vi "SRX_Read Quad Sensor Data.vi"(8 "Error":errorcluster, 11 "PhoenixMotorControlDevRef":T2) -> (0 "Error Out":errorcluster, 3 "Quad Sensor Data Out":T1)   [LabVIEW 2017]
uses:
  <vilib>/Rock Robotics/WPI/MotorControl/WPI_MotorControlDeviceRef.ctl
  <vilib>/Rock Robotics/WPI/MotorControl/WPI_MotorControlType.ctl
  <vilib>/Rock Robotics/SystemInterfaces/DIO/FPGA_DIOPWMChannel.ctl
  <vilib>/Rock Robotics/WPI/PWM/WPI_PWMDeadband.ctl
  <vilib>/Rock Robotics/SystemInterfaces/DIO/FPGA_DIOChannel.ctl
  TypeDefs SRX/Cluster_SRX_Sensor Quad Data.ctl
  System Drivers/Phoenix-LabVIEW/Motor Controller/Get/CTRE_Phoenix_MotorController_GetQuadPinData.vi
  System Drivers/Phoenix-LabVIEW/Motor Controller/Get/CTRE_Phoenix_MotorController_GetQuadratureData.vi
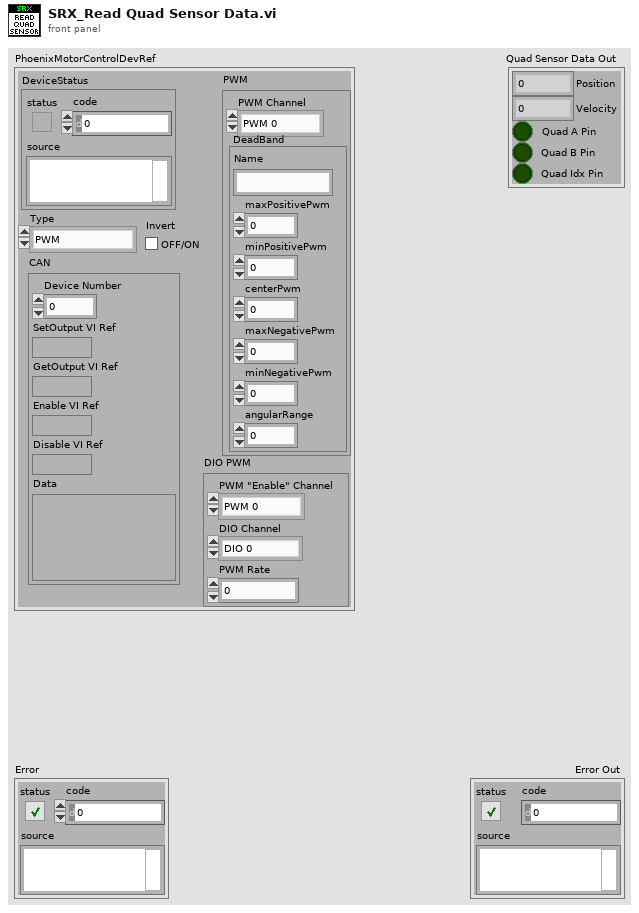
[diagram p1: front panel]
types:
  T1 = typedef "Cluster_SRX_Sensor Quad Data.ctl" = cluster{"Position":i32, "Velocity":i32, "Quad A Pin":bool, "Quad B Pin":bool, "Quad Idx Pin":bool}
  T2 = typedef "WPI_MotorControlDeviceRef.ctl" = cluster{"DeviceStatus":errorcluster, "Type":T3, "PWM":cluster{"PWM Channel":T4, "DeadBand":T5}, "CAN":cluster{"Device Number":u8, "SetOutput VI Ref":variant, "GetOutput VI Ref":variant, "Enable VI Ref":variant, "Disable VI Ref":variant, "Data":variant}, "Invert":bool, "DIO PWM":cluster{"PWM \"Enable\" Channel":T4, "DIOChannel":T6, "PWM Rate":dbl}}
  T3 = typedef "WPI_MotorControlType.ctl" = enum16{"PWM", "CAN", "DIO PWM"}
  T4 = typedef "FPGA_DIOPWMChannel.ctl" = enum8{"PWM 0", "PWM 1", "PWM 2", "PWM 3", "PWM 4", "PWM 5", "PWM 6", "PWM 7", "PWM 8", "PWM 9", "PWM MXP 0", "PWM MXP 1", "PWM MXP 2", "PWM MXP 3", "PWM MXP 4", "PWM MXP 5", "PWM MXP 6", "PWM MXP 7", "PWM MXP 8", "PWM MXP 9", "Invalid"}
  T5 = typedef "WPI_PWMDeadband.ctl" = cluster{"Name":string, "maxPositivePwm":i32, "minPositivePwm":i32, "centerPwm":i32, "maxNegativePwm":i32, "minNegativePwm":i32, "angularRange":u16}
  T6 = typedef "FPGA_DIOChannel.ctl" = enum8{"DIO 0", "DIO 1", "DIO 2", "DIO 3", "DIO 4", "DIO 5", "DIO 6", "DIO 7", "DIO 8", "DIO 9", "DIO MXP 0", "DIO MXP 1", "DIO MXP 2", "DIO MXP 3", "DIO MXP 4", "DIO MXP 5", "DIO MXP 6", "DIO MXP 7", "DIO MXP 8", "DIO MXP 9", "DIO MXP 10", "DIO MXP 11", "DIO MXP 12", "DIO MXP 13", "DIO MXP 14", "DIO MXP 15", "SPI Port CS1", "SPI Port CS2", "SPI Port CS3", "SPI Port MISO", "SPI Port MOSI", "Invalid"}
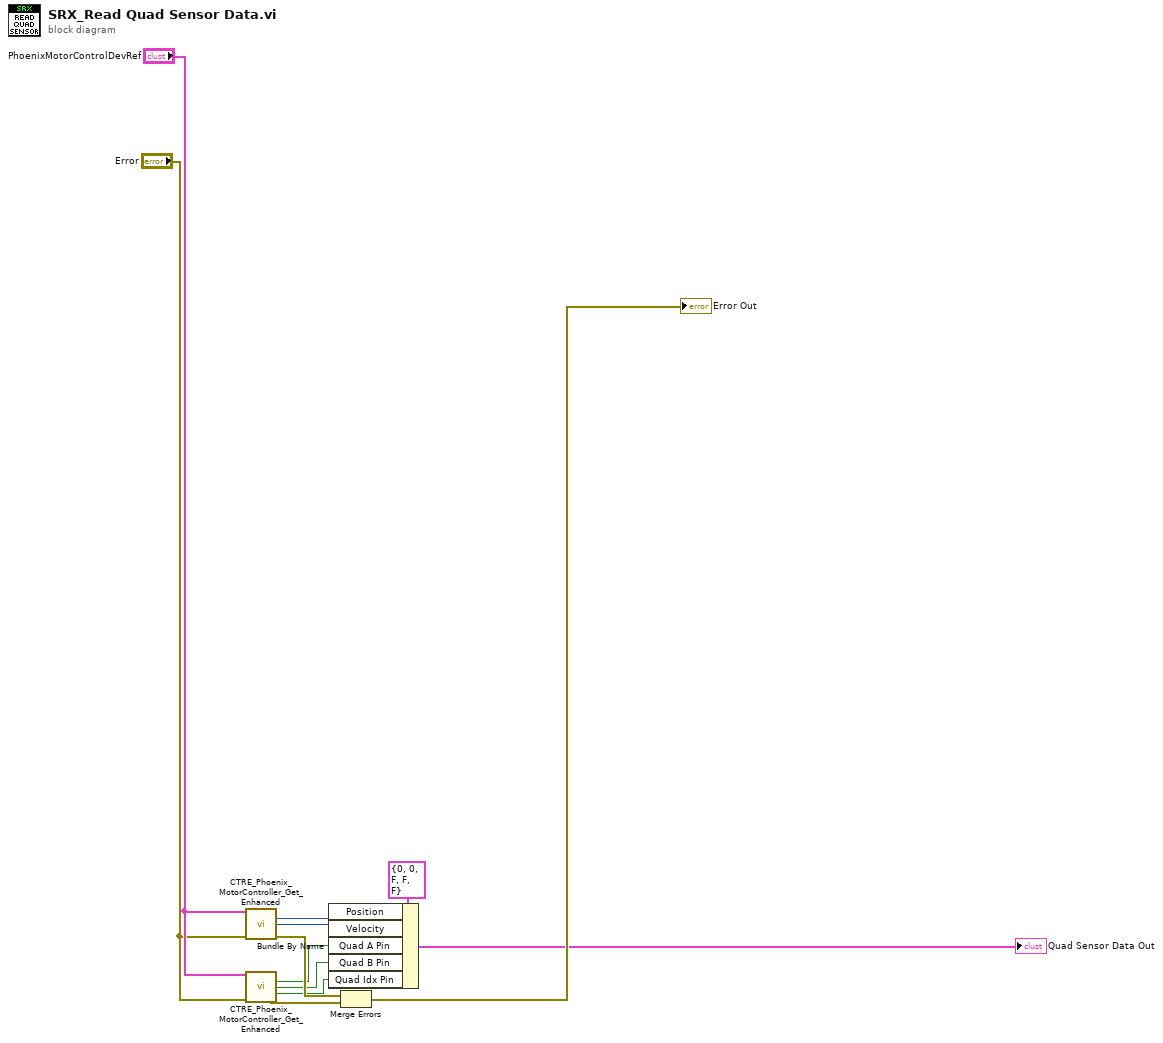
[diagram p0: block diagram]
diagram:
  n1 = call-poly "CTRE_Phoenix_MotorController_Get_Enhanced.vi"("PhoenixMotorControlDevRef"="PhoenixMotorControlDevRef", "error in"="Error") -> ("Quadrature Position"=w2:i32, "Quadrature Velocity"=w3:i32, "error out"=w9:errorcluster)  [unwired: 10 in, 1 out]
  n2 = call-poly "CTRE_Phoenix_MotorController_Get_Enhanced.vi"("PhoenixMotorControlDevRef"="PhoenixMotorControlDevRef", "error in"="Error") -> ("Quad A Pin"=w5:bool, "Quad B Pin"=w6:bool, "Quad Idx Pin"=w7:bool, "error out"=w8:errorcluster)  [unwired: 9 in, 1 out]
  n3 = Bundle By Name(cluster=T1 {"Position"=0, "Velocity"=0, "Quad A Pin"=FALSE, "Quad B Pin"=FALSE, "Quad Idx Pin"=FALSE} ("Quad Sensor Data"), "Position"=w2, "Velocity"=w3, "Quad A Pin"=w5, "Quad B Pin"=w6, "Quad Idx Pin"=w7) -> (→"Quad Sensor Data Out":T1)
  n4 = Merge Errors(w9, w8) -> (→"Error Out":errorcluster)
